vi "reset_final.vi"() -> ()   [LabVIEW 2017]
panel:
  in  "String":string
  in  "SoftTrigger":bool=TRUE
  in  "address":string="192.168.10.35"
  in  "error in (no error)":errorcluster
  out "error out":errorcluster
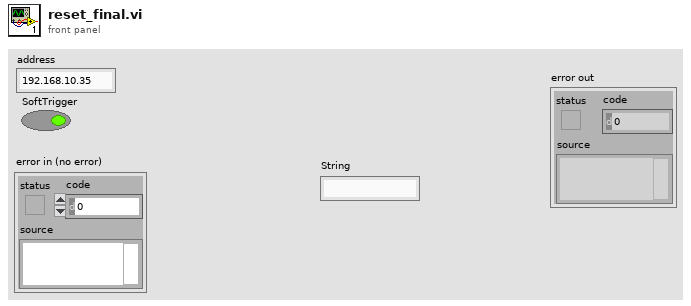
[diagram p1: front panel]
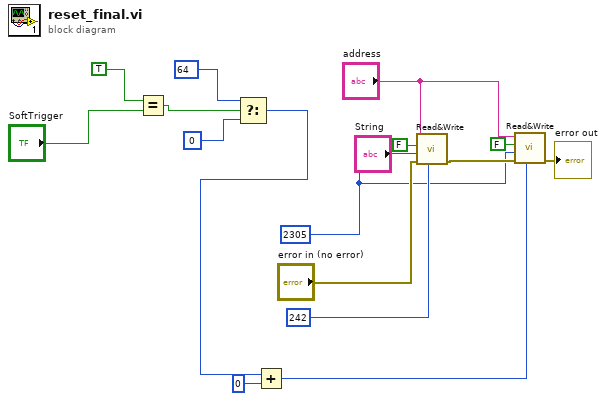
[diagram p0: block diagram]
diagram:
  w9 = u32 2305 ("Address")
  n1 = Equal?(x=TRUE, y="SoftTrigger") -> (x = y?=w7:bool)
  n2 = Select(t=u8 64 ("In 3"), s=w7, f=u8 0 ("In 3")) -> (s? t:f=w2:u8)
  n3 = Add(x=w2, y=u8 0) -> (x+y=w3:u8)
  n4 = call "Read&Write.vi"("In"=u8 242, "error in (no error)"="error in (no error)", "Address"=w9, "Read (TRUE)"=FALSE, "address"="address") -> ("error out"=w16:errorcluster)  [unwired: 5 in, 1 out]
  n5 = call "Read&Write.vi"("In"=w3, "error in (no error)"=w16, "Address"=w9, "Read (TRUE)"=FALSE, "address"="address") -> ("error out"=→"error out":errorcluster)  [unwired: 5 in, 1 out]
